vi "Main_05A.vi"() -> ()   [LabVIEW 2025]
uses:
  Utility/Universal Utility/TypeDefs_Utility/Cluster_Row-Column.ctl
  9e3f57c0-2ef8-4495-8287-c6a42a5fb955.vi
  Utility/Universal Utility/TypeDefs_Utility/ENUM_4 Directions U-D-L-R.ctl
  Utility/Universal Utility/TypeDefs_Utility/ENUM_8 Directions U-D-L-R.ctl
panel:
  out "Array":u64[](array[numeric])
  out "x-1":u64
  out "MATCH":bool
  in  "Select Data":enum32{"Example", "Puzzle"}(tab)
  in  "EX Target":u32=3
  in  "Example":string="3-5\n10-14\n16-20\n12-18\n\n1\n5\n8\n11\n17\n32"
  in  "Puzzle":string="505104443555011-505832008521290\n183705568221799-189071596736306\n25714421842394-26498060657296\n324591982604436-326326266144576\n194954655268286-199771011784310\n32539515377401-39552166142220\n326326266144577-330576407995732\n45877724695638-45877724695638\n245990755269494-248893742631986\n316826876448244-321016747706186\n23726069480801-24221552311396\n282687875186245-282687875186245\n84944235636755-86138442862850\n27463398169403-27981167005022\n388889831860114-389071080230049\n178876097666360-180498038018267\n509753176570993-510393291709325\n137682268842164-139478866740539\n504458187396917-505104443555011\n5030..."
  in  "Puzzle Target":u32
  out "Answer":u32
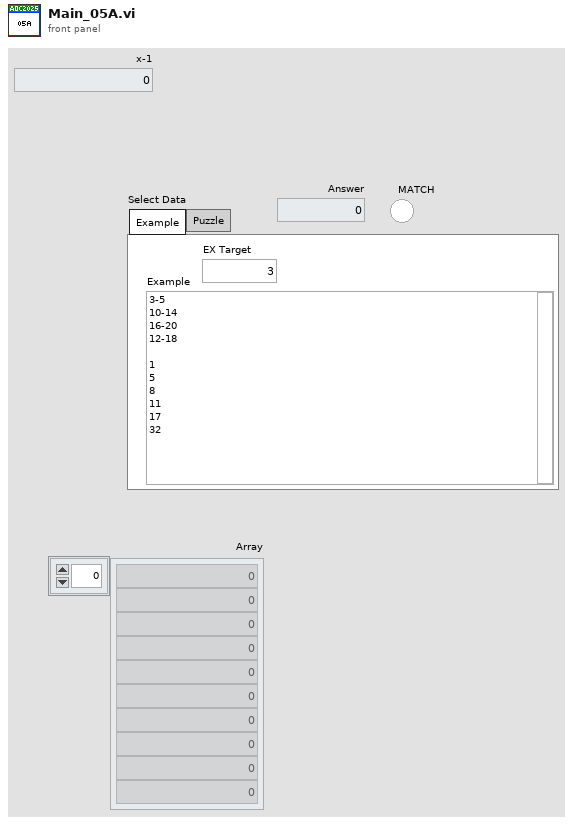
[diagram p1: front panel]
types:
  T1 = typedef "ENUM_8 Directions U-D-L-R.ctl" = enum16{"Up;-1,0", "Up-Right;-1,1", "Right;0,1", "Down-Right;1,1", "Down;1,0", "Down-Left;1,-1", "Left;0,-1", "Up-Left;-1,-1"}
  T2 = typedef "ENUM_4 Directions U-D-L-R.ctl" = enum16{"Up;-1,0", "Right;0,1", "Down;1,0", "Left;0,-1"}
  T3 = typedef "Cluster_Row-Column.ctl" = cluster{"R":i32, "C":i32}
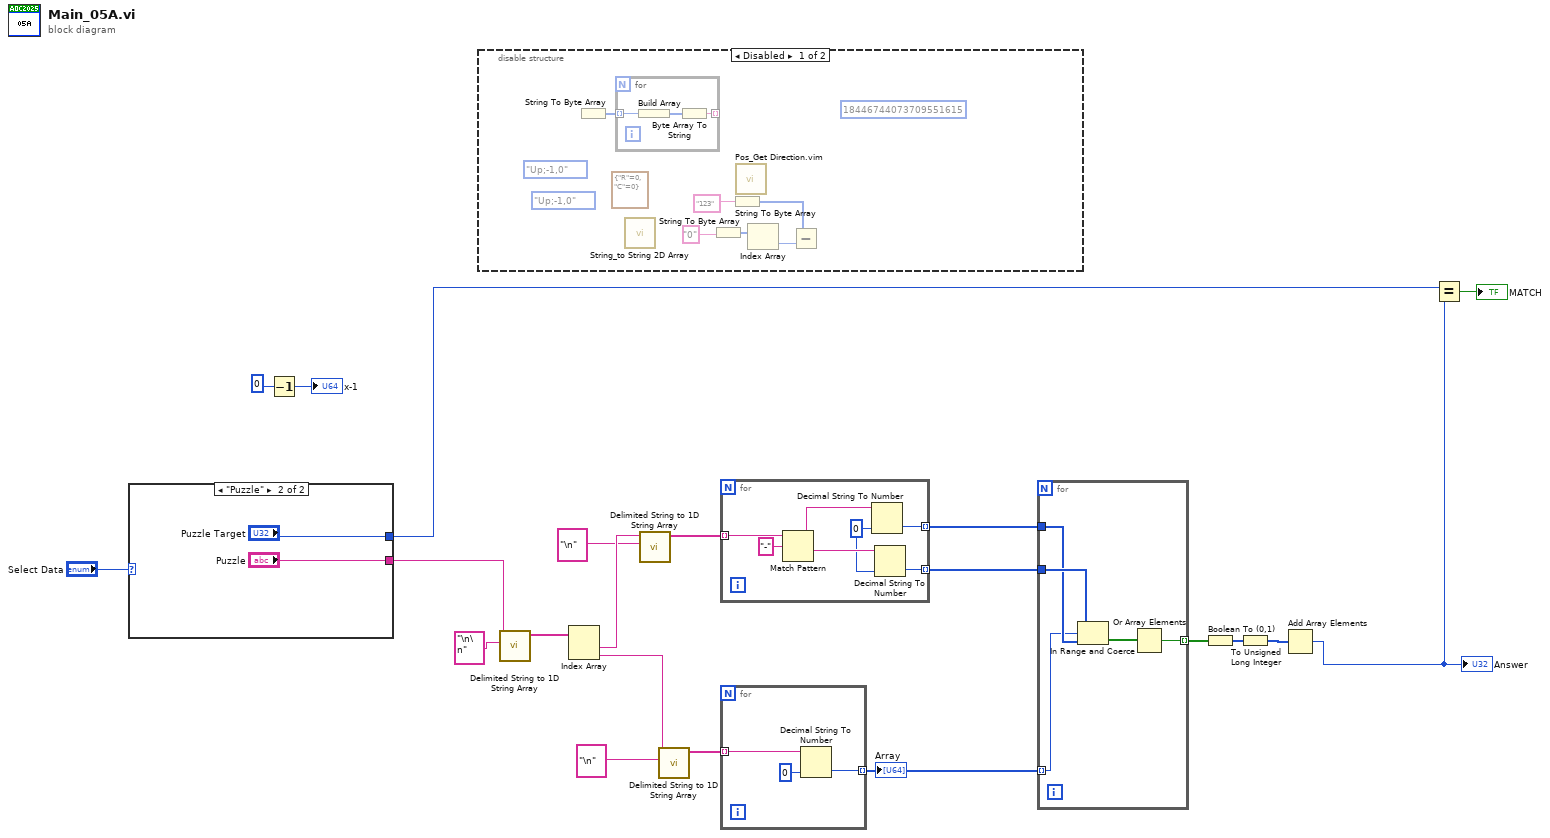
[diagram p0: block diagram]
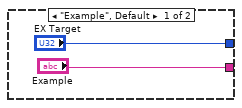
[diagram p2: hidden frame]
diagram:
  n1 = case shown="\"Puzzle\"" "Select Data" {
    tunnel: ["Example" "Puzzle"] -> w20
    tunnel: ["EX Target" "Puzzle Target"] -> w17
    frame "Example", Default {
    }
    frame "Puzzle" {
    }
  }
  n2 = Decrement(x=u64 0) -> (x-1=→"x-1":u64)
  n3 = disable-structure shown="Disabled" {
    frame Disabled {
      (unwired) u64 18446744073709551615 ("x-1")
      (unwired) ENUM_8_Directions_U-D-L-R."Up;-1,0" ("Direction 8")
      (unwired) ENUM_4_Directions_U-D-L-R."Up;-1,0" ("Direction")
      (unwired) T3 {"R"=0, "C"=0} ("Position")
      n4 = String To Byte Array() -> (unsigned byte array=w26:u8[])  [unwired: 1 in]
      n5 = for {
        tunnel: w26 -> [w34] mode=indexing
        tunnel: [w32] -> _ mode=indexing
        n6 = Build Array(w34) -> (w33:u8[])
        n7 = Byte Array To String(unsigned byte array=w33) -> (string=w32:string)
      }
      n8 = call "String_to String 2D Array.vi"() -> ()  [unwired: 11 in, 1 out]
      n9 = String To Byte Array(string="0") -> (unsigned byte array=w29:u8[])
      n10 = String To Byte Array(string="123") -> (unsigned byte array=w27:u8[])
      n11 = call "Pos_Get Direction.vim"() -> ()  [unwired: 11 in, 1 out]
      n12 = Index Array(array=w29) -> (element=w28:u8)  [unwired: 1 in]
      n13 = Subtract(x=w27, y=w28) -> ()  [unwired: 1 out]
    }
    frame Enabled {
    }
  }
  n14 = call <vilib>:"Delimited String to 1D String Array.vi"("delimiter"="\n\n" ("delimiter (Tab)"), "delimited string"=w20) -> ("string array"=w14:string[])  [unwired: 9 in]
  n15 = Index Array(array=w14) -> (element #1=w13:string, element #2=w10:string)  [unwired: 2 in]
  n16 = call <vilib>:"Delimited String to 1D String Array.vi"("delimiter"="\n" ("delimiter (Tab)"), "delimited string"=w13) -> ("string array"=w8:string[])  [unwired: 9 in]
  n17 = call <vilib>:"Delimited String to 1D String Array.vi"("delimiter"="\n" ("delimiter (Tab)"), "delimited string"=w10) -> ("string array"=w9:string[])  [unwired: 9 in]
  n18 = for {
    tunnel: w8 -> [w41] mode=indexing
    tunnel: [w37] -> w5 mode=indexing
    tunnel: [w35] -> w7 mode=indexing
    w36 = u64 0 ("default (0 I32)")
    n19 = Match Pattern(string=w41, regular expression="-") -> (before substring=w39:string, after substring=w38:string)  [unwired: 1 in, 2 out]
    n20 = Decimal String To Number(string=w39, default (0L)=w36) -> (number=w35:u64)  [unwired: 1 in, 1 out]
    n21 = Decimal String To Number(string=w38, default (0L)=w36) -> (number=w37:u64)  [unwired: 1 in, 1 out]
  }
  n22 = for {
    tunnel: w9 -> [w44] mode=indexing
    tunnel: [w42] -> w6 mode=indexing
    n23 = Decimal String To Number(string=w44, default (0L)=u64 0 ("default (0 I32)")) -> (number=w42:u64)  [unwired: 1 in, 1 out]
  }
  "Array" <- w6
  n24 = for {
    tunnel: w7 -> [w48]
    tunnel: w6 -> [w47] mode=indexing
    tunnel: w5 -> [w49]
    tunnel: [w45] -> w4 mode=indexing
    n25 = In Range and Coerce(upper limit=w49, x=w47, lower limit=w48) -> (In Range?=w46:bool[])  [unwired: 1 out]
    n26 = Or Array Elements(Boolean array=w46) -> (logical OR=w45:bool)
  }
  n27 = Boolean To (0,1)(Boolean=w4) -> (0, 1=w3:i16[])
  n28 = To Unsigned Long Integer(number=w3) -> (unsigned 32bit integer=w1:u32[])
  n29 = Add Array Elements(numeric array=w1) -> (sum=w2:u32)
  "Answer" <- w2
  n30 = Equal?(x=w17, y=w2) -> (x = y?=→"MATCH":bool)
